vi "EIP_data generator.vi"() -> ()   [LabVIEW 2023]
doc: "Demonstrates how to read and set the attributes of Identity Object using Explicit Messaging."
uses:
  <vilib>/ethernetip/ethernetip.llb/EthernetIPAssemblyType.ctl
  <vilib>/ethernetip/ethernetip.lvlib
panel:
  out "Array":sgl[](array[numeric])
  in  "Size (bytes)":u32=32
  in  "update rate [ms]":u32=500
  in  "stop":bool
  out "running?":bool
  in  "timeout [ms]":i32=1000
  in  "instance":u32=1
  # "Configuration"
  # "Original Attribute Values"
  # "Assign Attribute Values"
  # "Assigned Attribute Values"
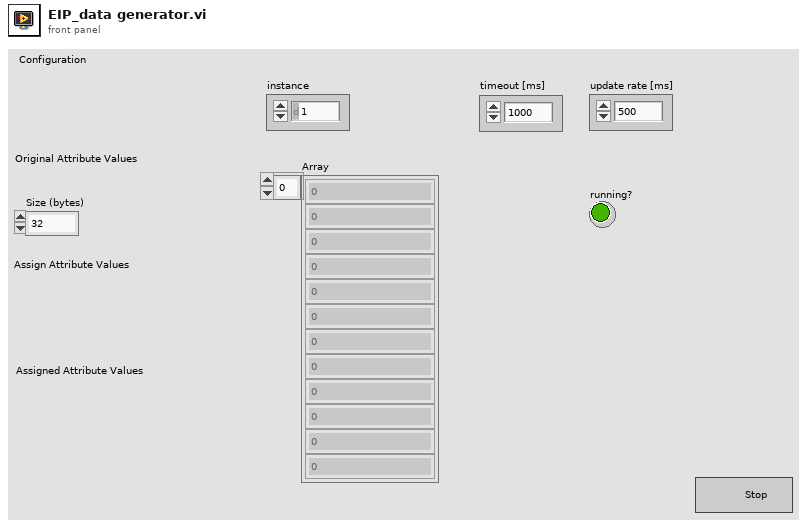
[diagram p1: front panel]
types:
  T1 = typedef "ethernetip.lvlib/EthernetIPAssemblyType.ctl" = enum16{"Producing", "Consuming", "Configuration"}
  T2 = typedef "ethernetip.lvlib/ethernetip.ctl" = refnum<k21>
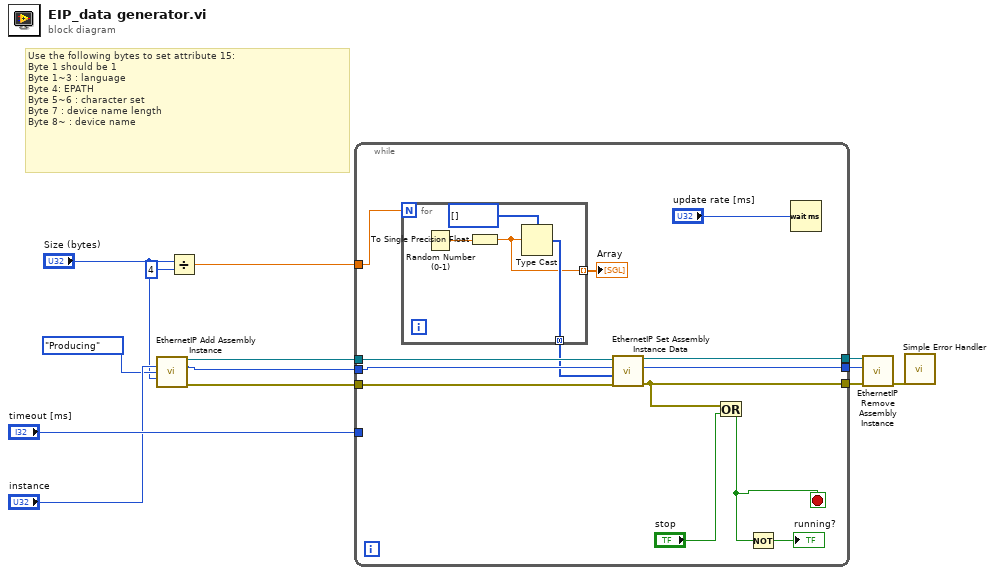
[diagram p0: block diagram]
diagram:
  # "Use the following bytes to set attribute 15:\nByte 1 should be 1\nByte 1~3 : language\nByte 4: EPATH\nByte 5~6 : character set\nByte 7 : device name length\nByte 8~ : device name"
  n1 = call <vilib>:"EthernetIP Add Assembly Instance.vi"("Instance ID in"="instance", "Type"=EthernetIPAssemblyType."Producing", "Size (bytes)"="Size (bytes)") -> ("Session out"=w11:T2, "Instance ID out"=w10:u32, "error out"=w12:errorcluster)  [unwired: 2 in, 8 out]
  n2 = Divide(x="Size (bytes)", y=u32 4) -> (x/y=w1:dbl)
  n3 = while {
    tunnel: "timeout [ms]" -> [_]
    tunnel: w12 -> [w22]
    tunnel: w11 -> [w21]
    tunnel: w10 -> [w20]
    tunnel: [w19] -> w9
    tunnel: [w18] -> w8
    tunnel: [w17] -> w7
    tunnel: w1 -> [w16]
    stop <- w23 stop-if-true
    n4 = for {
      N: w16 -> [_]
      tunnel: [w28] -> w15 mode=concatenating
      tunnel: [w27] -> w14 mode=indexing
      n5 = Random Number (0-1)() -> (number: 0 to 1=w30:dbl)
      n6 = To Single Precision Float(number=w30) -> (single precision float=w27:sgl)
      n7 = Type Cast(type=u8[] [] ("reversed array"), x=w27) -> (*(type *) &x=w28:u8[])
    }
    "Array" <- w14
    n8 = call <vilib>:"EthernetIP Set Assembly Instance Data.vi"("error in"=w22, "Data"=w15, "Instance ID in"=w20, "Session in"=w21) -> ("error out"=w17:errorcluster, "Instance ID out"=w19:u32, "Session out"=w18:T2)  [unwired: 5 out]
    n9 = Or(x=w17, y="stop") -> (x .or. y?=w23:bool)
    n10 = Not(x=w23) -> (.not. x?=→"running?":bool)
    n11 = Wait (ms)(milliseconds to wait="update rate [ms]") -> ()  [unwired: 1 out]
  }
  n12 = call <vilib>:"EthernetIP Remove Assembly Instance.vi"("Session in"=w8, "Instance ID"=w9, "error in"=w7) -> ("error out"=w4:errorcluster)  [unwired: 12 out]
  n13 = call <vilib>:"Simple Error Handler.vi"("error in (no error)"=w4) -> ()  [unwired: 1 in, 8 out]
